vi "Dashboard and Primary Interface.vi"() -> ()   [LabVIEW 2021]
uses:
  Z:/Samples/LabVIEW/Library/UnderAutomation.UniversalRobots.dll
  Library/UnderAutomation.UniversalRobots.dll
panel:
  out "Powered on":bool
  in  "Script to execute":string
  in  "Send script":bool
  out "Z":dbl
  out "Y":dbl
  out "X":dbl
  in  "Robot IP":string
  out "Connect error":errorcluster
  in  "Power off":bool
  in  "Power on\nRelease brake":bool
  out "Connected":bool
  out "License state":string
  in  "Connect":bool
  # "1. Connect to the robot"
  # "2. Dashboard"
  # "3. Primary Interface"
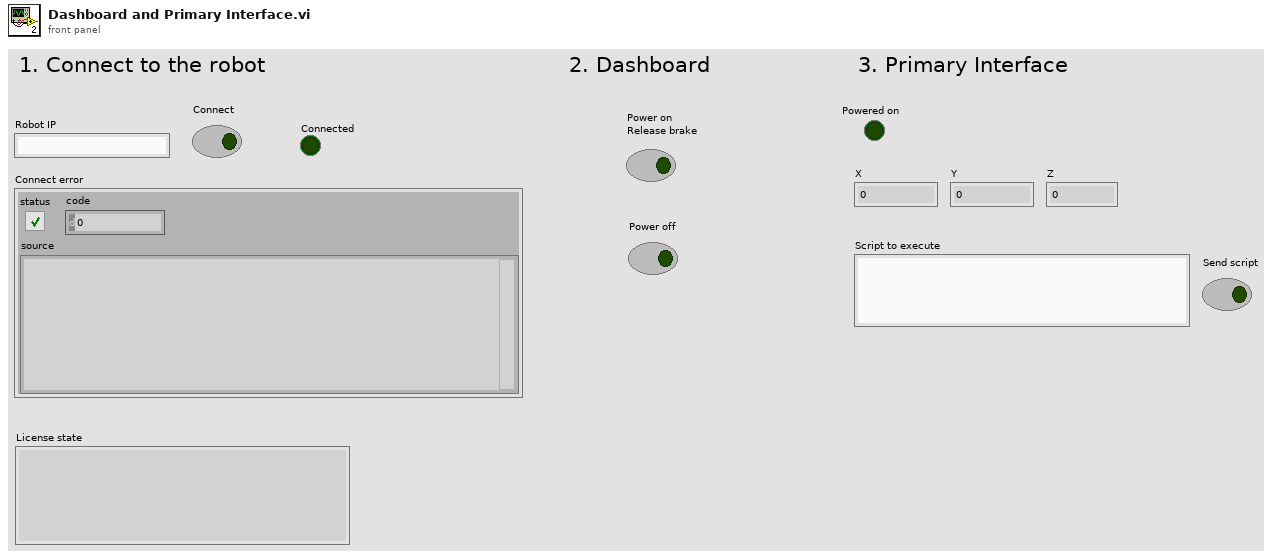
[diagram p1: front panel]
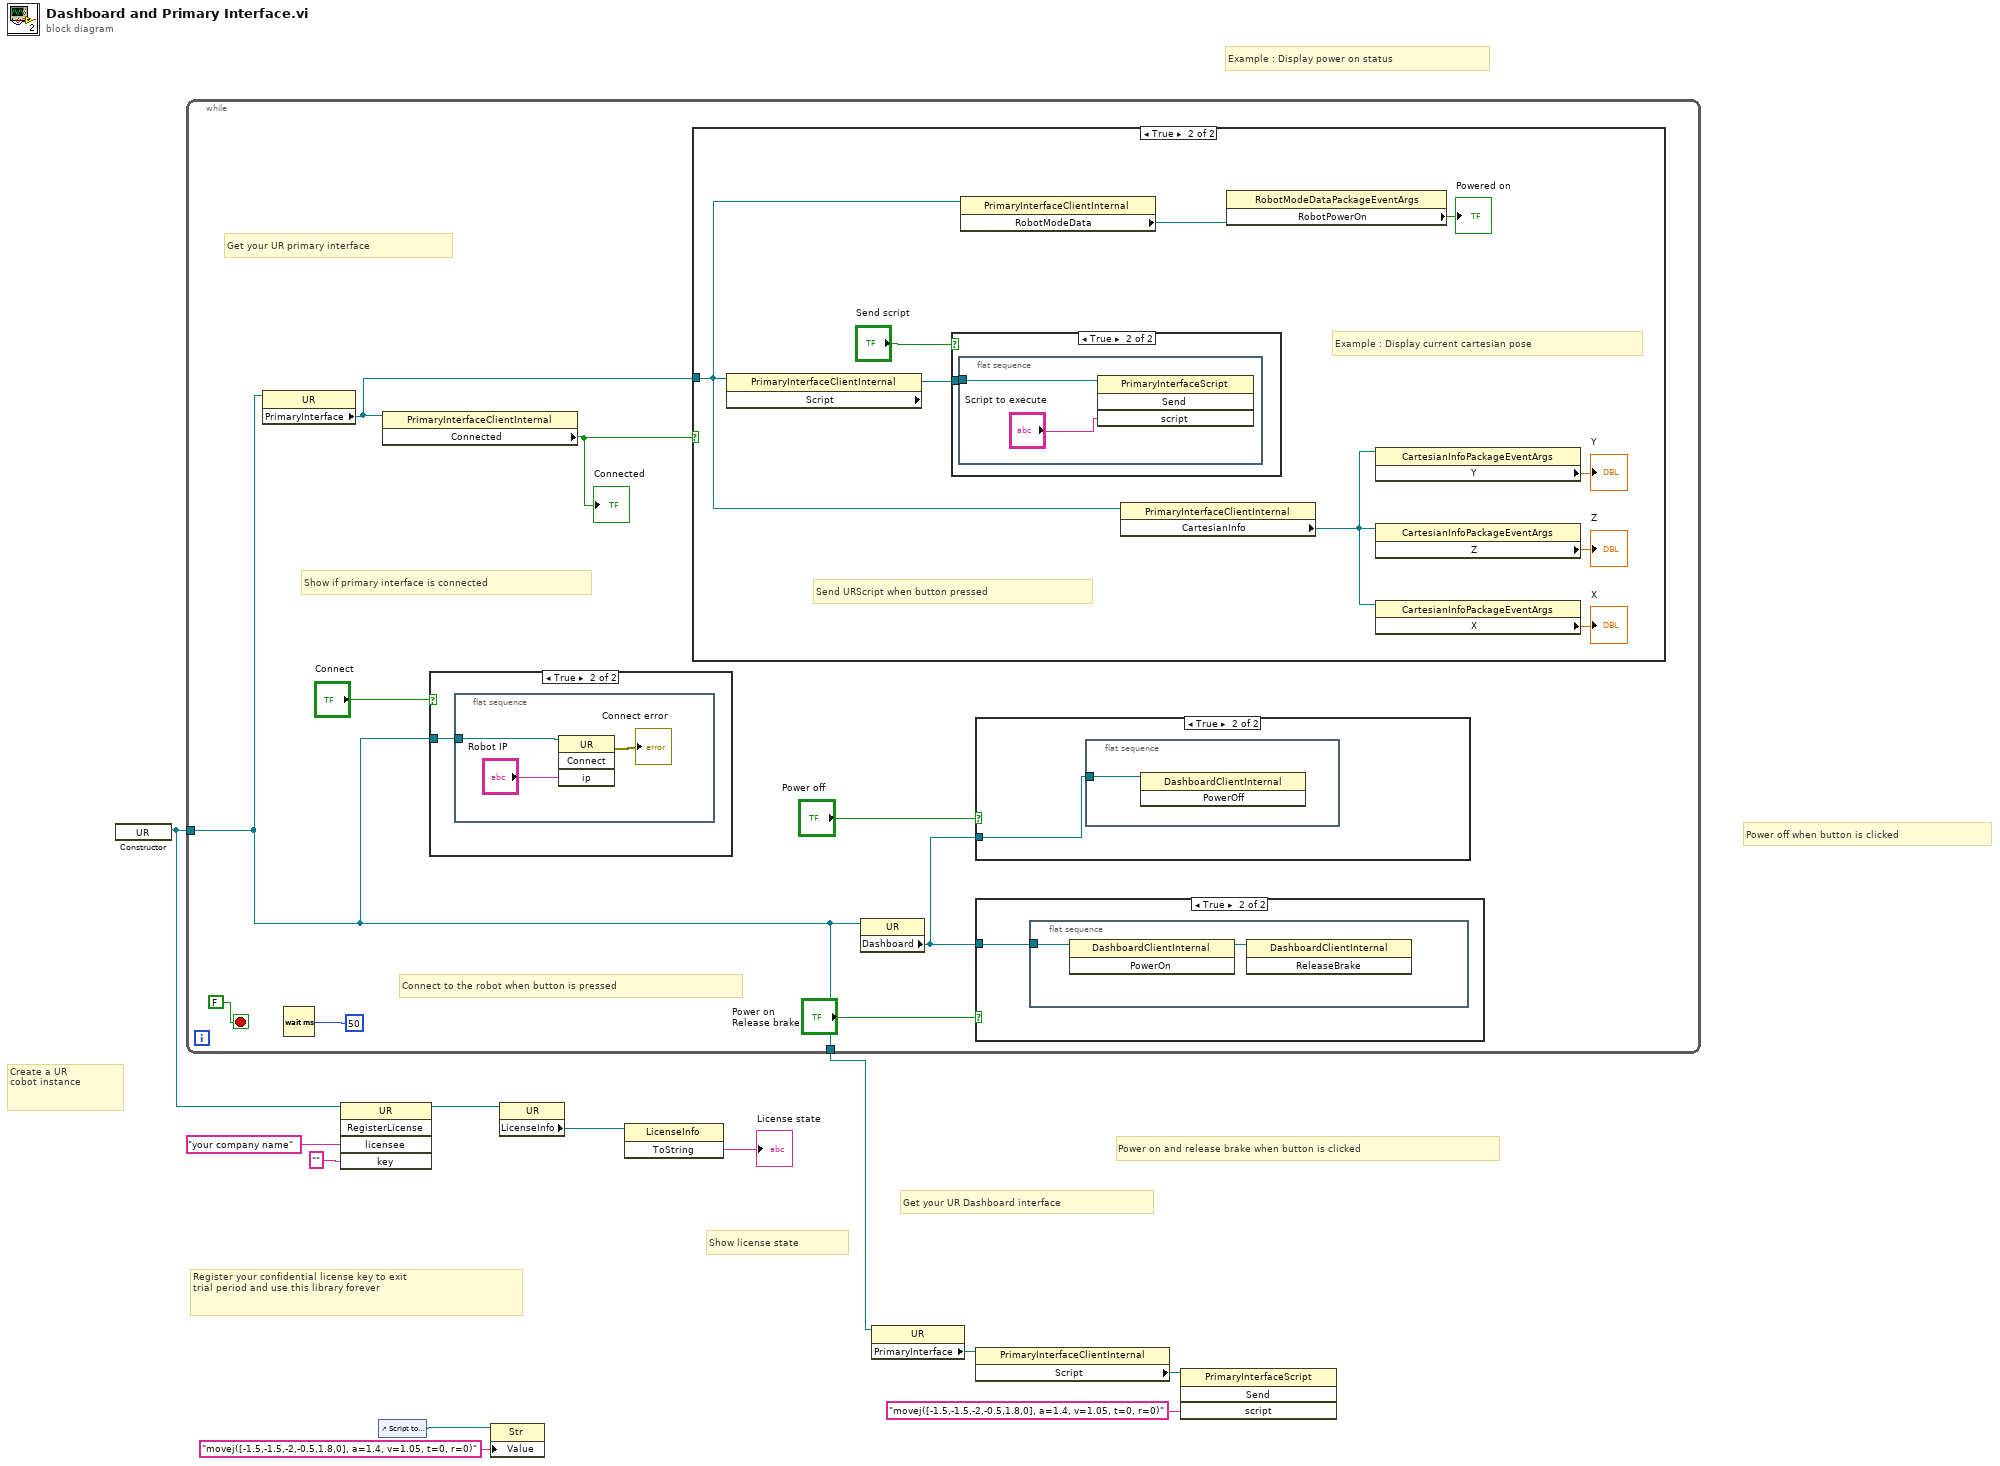
[diagram p0: block diagram]
diagram:
  # "Example : Display power on status"
  # "Create a UR\ncobot instance"
  # "Show license state"
  # "Register your confidential license key to exit\ntrial period and use this library forever"
  # "Power off when button is clicked"
  # "Power on and release brake when button is clicked"
  # "Get your UR Dashboard interface"
  n1 = constructor class="UR"() -> (reference out=w7:refnum<k24>)  [unwired: 3 in, 2 out]
  n2 = while {
    tunnel: w7 -> [w13]
    tunnel: [w13] -> w1
    stop <- FALSE stop-if-true
    # "Connect to the robot when button is pressed"
    # "Show if primary interface is connected"
    # "Get your UR primary interface"
    n3 = property class="UR"(reference=w13) -> ("PrimaryInterface"=w16:refnum<k24>)  [unwired: 1 in, 2 out]
    n4 = Wait (ms)(milliseconds to wait=u32 50) -> ()  [unwired: 1 out]
    n5 = property class="PrimaryInterfaceClientInternal"(reference=w16) -> ("Connected"=w15:bool)  [unwired: 1 in, 2 out]
    "Connected" <- w15
    n6 = case shown="True" "Connect" {
      tunnel: w13 -> [_ w39]
      frame False {
      }
      frame True {
        n7 = flat-sequence {
          tunnel: w39 -> [w41]
          frame #0 {
            n8 = invoke class="UR" method="Connect"(reference=w41, "ip"="Robot IP") -> (error out=→"Connect error":errorcluster)  [unwired: 2 in, 3 out]
          }
        }
      }
    }
    n9 = case shown="True" w15 {
      tunnel: w16 -> [_ w22]
      frame False {
      }
      frame True {
        # "Send URScript when button pressed"
        # "Example : Display current cartesian pose"
        n10 = property class="PrimaryInterfaceClientInternal"(reference=w22) -> ("Script"=w29:refnum<k24>)  [unwired: 1 in, 2 out]
        n11 = case shown="True" "Send script" {
          tunnel: w29 -> [_ w31]
          frame False {
          }
          frame True {
            n12 = flat-sequence {
              tunnel: w31 -> [w33]
              frame #0 {
                n13 = invoke class="PrimaryInterfaceScript" method="Send"(reference=w33, "script"="Script to execute") -> ()  [unwired: 2 in, 4 out]
              }
            }
          }
        }
        n14 = property class="PrimaryInterfaceClientInternal"(reference=w22) -> ("RobotModeData"=w28:refnum<k24>)  [unwired: 1 in, 2 out]
        n15 = property class="PrimaryInterfaceClientInternal"(reference=w22) -> ("CartesianInfo"=w23:refnum<k24>)  [unwired: 1 in, 2 out]
        n16 = property class="RobotModeDataPackageEventArgs"(reference=w28) -> ("RobotPowerOn"=→"Powered on":bool)  [unwired: 1 in, 2 out]
        n17 = property class="CartesianInfoPackageEventArgs"(reference=w23) -> ("Y"=→"Y":dbl)  [unwired: 1 in, 2 out]
        n18 = property class="CartesianInfoPackageEventArgs"(reference=w23) -> ("Z"=→"Z":dbl)  [unwired: 1 in, 2 out]
        n19 = property class="CartesianInfoPackageEventArgs"(reference=w23) -> ("X"=→"X":dbl)  [unwired: 1 in, 2 out]
      }
    }
    n20 = property class="UR"(reference=w13) -> ("Dashboard"=w17:refnum<k24>)  [unwired: 1 in, 2 out]
    n21 = case shown="True" "Power off" {
      tunnel: w17 -> [_ w34]
      frame False {
      }
      frame True {
        n22 = flat-sequence {
          tunnel: w34 -> [w35]
          frame #0 {
            n23 = invoke class="DashboardClientInternal" method="PowerOff"(reference=w35) -> ()  [unwired: 2 in, 3 out]
          }
        }
      }
    }
    n24 = case shown="True" "Power on\nRelease brake" {
      tunnel: w17 -> [_ w36]
      frame False {
      }
      frame True {
        n25 = flat-sequence {
          tunnel: w36 -> [w38]
          frame #0 {
            n26 = invoke class="DashboardClientInternal" method="PowerOn"(reference=w38) -> (reference out=w37:refnum<k24>)  [unwired: 2 in, 2 out]
            n27 = invoke class="DashboardClientInternal" method="ReleaseBrake"(reference=w37) -> ()  [unwired: 2 in, 3 out]
          }
        }
      }
    }
  }
  n28 = invoke class="UR" method="RegisterLicense"(reference=w7, "licensee"="your company name", "key"="") -> (reference out=w9:refnum<k24>)  [unwired: 2 in, 4 out]
  n29 = control-ref of="Script to execute"() -> (w6:refnum<vi>)
  n30 = property class="Str"(reference=w6, "Value"="movej([-1.5,-1.5,-2,-0.5,1.8,0], a=1.4, v=1.05, t=0, r=0)") -> ()  [unwired: 1 in, 2 out]
  n31 = property class="UR"(reference=w9) -> ("LicenseInfo"=w8:refnum<k24>)  [unwired: 1 in, 2 out]
  n32 = invoke class="LicenseInfo" method="ToString"(reference=w8) -> ("ToString"=→"License state":string)  [unwired: 2 in, 2 out]
  n33 = property class="UR"(reference=w1) -> ("PrimaryInterface"=w2:refnum<k24>)  [unwired: 1 in, 2 out]
  n34 = property class="PrimaryInterfaceClientInternal"(reference=w2) -> ("Script"=w4:refnum<k24>)  [unwired: 1 in, 2 out]
  n35 = invoke class="PrimaryInterfaceScript" method="Send"(reference=w4, "script"="movej([-1.5,-1.5,-2,-0.5,1.8,0], a=1.4, v=1.05, t=0, r=0)" ("Value")) -> ()  [unwired: 2 in, 4 out]
